vi "calibrationElectrometer_logEvent_SettingsAppliedSerialConfiguration.vi"(8 "error in (no error)":errorcluster, 11 "logevent_SettingsApplied_SerialConfiguration_Ctl":T1) -> (0 "error out":errorcluster, 2 "function return":i32, 3 "logevent_SettingsApplied_SerialConfiguration_Ctl out":T1)   [LabVIEW 2016, in "SALLV_calibrationElectrometer.lvlib"]
doc: "int calibrationElectrometer_shm_logEvent_SettingsApplied_SerialConfigurationLV(calibrationElectrometer_logevent_SettingsApplied_SerialConfigurationLV *logevent_SettingsApplied_SerialConfiguration_Ctl );"
uses:
  SALLV_calibrationElectrometer.lvlib
  DataTypes/logevent_SettingsApplied_SerialConfiguration.ctl
  SALLV_calibrationElectrometer.so
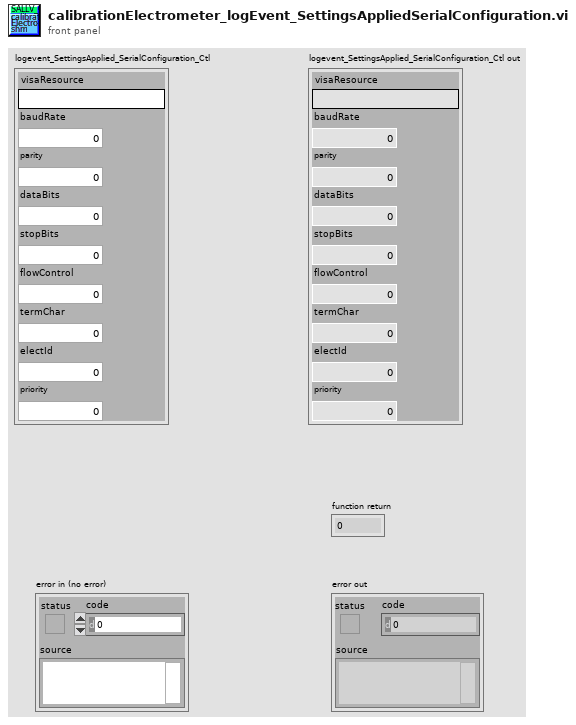
[diagram p1: front panel]
types:
  T1 = typedef "SALLV_calibrationElectrometer.lvlib/logevent_SettingsApplied_SerialConfiguration.ctl" = cluster{"visaResource":string, "baudRate":i32, "parity":i32, "dataBits":i32, "stopBits":i32, "flowControl":i32, "termChar":i32, "electId":i16, "priority":i32}
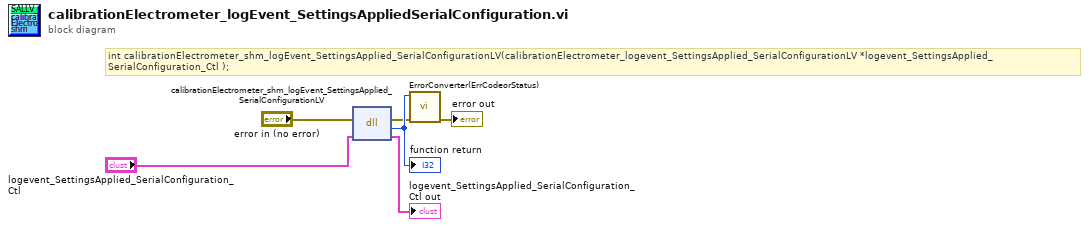
[diagram p0: block diagram]
diagram:
  # "int calibrationElectrometer_shm_logEvent_SettingsApplied_SerialConfigurationLV(calibrationElectrometer_logevent_SettingsApplied_SerialConfigurationLV *logevent_SettingsApplied_SerialConfiguration_Ctl );"
  n1 = dll-call lib="home/andres/Desktop/SAL_calibrationElectrometer/SALLV_calibrationElectrometer.*" fn="calibrationElectrometer_shm_logEvent_SettingsApplied_SerialConfigurationLV"(error in="error in (no error)", "logevent_SettingsApplied_SerialConfiguration_Ctl"="logevent_SettingsApplied_SerialConfiguration_Ctl") -> (error out=w2:errorcluster, w6:i32, "logevent_SettingsApplied_SerialConfiguration_Ctl"=→"logevent_SettingsApplied_SerialConfiguration_Ctl out":T1)  [unwired: 2 in, 1 out]
  "function return" <- w6
  n2 = call "ErrorConverter(ErrCodeorStatus).vi"("error in (no error)"=w2, "error code"=w6) -> ("error out"=→"error out":errorcluster)  [unwired: 9 in]
